vi "Shooter Control wPID.vi"() -> (7 "Robot Values Output":T1={"Robot Drive"={"Left Motor Power"=0.0, "Right Motor Power"=0.0, "Left Encoder Value"=0.0, "Right Encoder Value"=0.0, "High Gear?"=FALSE, "PTO?"=FALSE}, "Sensors"={"Gyro Angle"=0, "Recalibrate Gyro"=FALSE, "Reset Gyro"=FALSE, "Ultrasonic"=0.0}, "Shooter"={"Prep Wheels"=FALSE, "Shoot"=FALSE, "Left Shooter Wheel Speed"=0.0, "Wheels Moving"=FALSE, "Shooter Prepped"=FALSE, "Shooter RPS SP"=0.0, "Shooting?"=FALSE, "Left Shooter Wheel Power"=0.65, "Right Shooter Wheel Power"=0.0, "Acquisition Conveyor Power"=0.0, "Hopper Beater Bar Power"=0.0, "Filtered Left Shooter Speed"=0.0, "Acquisition Motor Power"=0.0, "Joystick Add"=0.0, "D-Pad Add"=0.0, "Shooter Use PID?"=FALSE}, "Robot States"={"Drive mode"="", "Alliance"=enum."Red", "Position"=enum."1"}, "Gear"={"Ejection Active"=FALSE}})   [LabVIEW 2016]
uses:
  Robot Values.ctl
  <vilib>/Rock Robotics/WPI/DriverStation/WPI_DriverStationAllianceInfo.ctl
  <vilib>/Rock Robotics/WPI/DriverStation/WPI_DriverStationPositionInfo.ctl
  <vilib>/Rock Robotics/Network Tables/NT Read Number.vi
  Robot Values.vi
  <vilib>/addons/control/pid/pid.llb/PID (DBL).vi
  LED Send Global.vi
  <vilib>/addons/control/pid/NI_PID_pid.lvlib
  <vilib>/ptbypt/NI_PtbyPt.lvlib
panel:
  in  "Feeder SP":dbl=0.88 format="%#_13g"
  out "Offset time":timestamp
  in  "Time Target In":dbl=0.6 caption="Time Target (s)"
  in  "Time Target Out":dbl caption="Time Target (s)"
  in  "Tolerance":dbl=2.0 format="%#_13g"
  in  "output range":cluster{"output high":dbl, "output low":dbl}={"output high"=0.049999999999999996, "output low"=-0.04999999999999999}
  in  "Agitate State":enum16{"In", "Out"}(ring)
  in  "Feeder Out SP":dbl=0.6
  in  "Feeder In SP":dbl=0.6
  out "Baseline Power":dbl=0.75 format="%#_13g"
  in  "Time Tolerance (s)":dbl=0.15 format="%#_13g"
  in  "PID gains":T4={"proportional gain (Kc)"=20.0, "integral time (Ti, min)"=0.010000000000000002, "derivative time (Td, min)"=0.0} {"derivative time (Td, min)" format="%.3f"; "integral time (Ti, min)" format="%.3f"; "proportional gain (Kc)" format="%.3f"}
  out "setpoint":dbl=39.0 format="%#_13g"
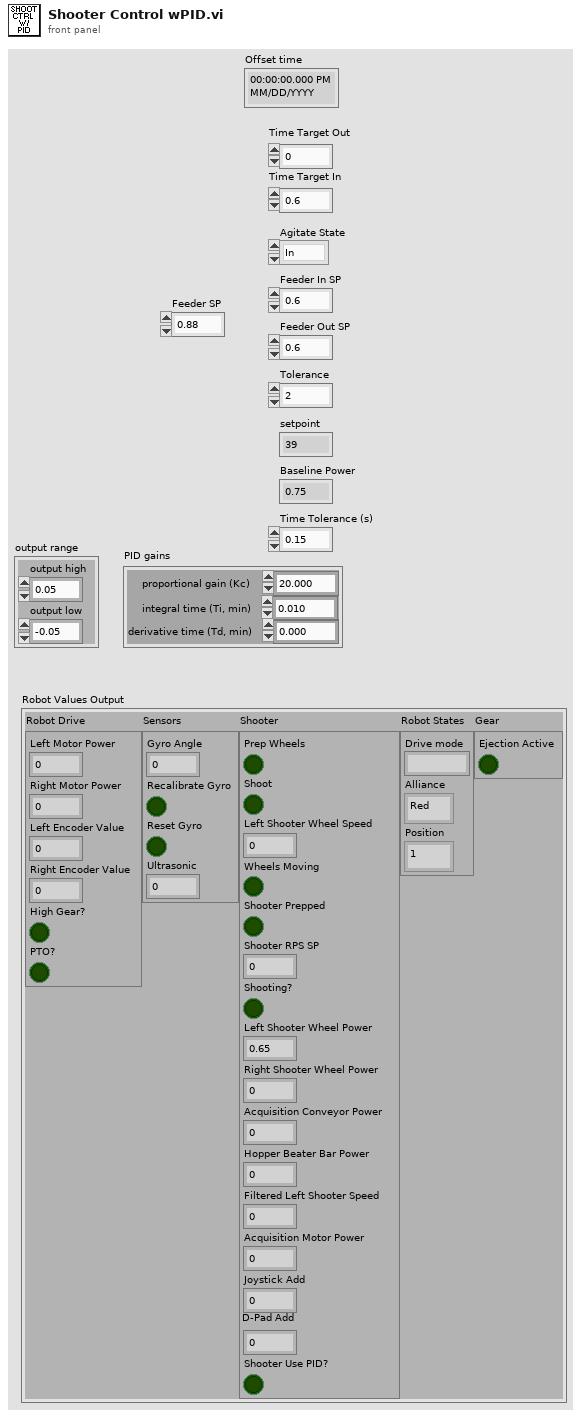
[diagram p1: front panel]
types:
  T1 = typedef "Robot Values.ctl" = cluster{"Robot Drive":cluster{"Left Motor Power":dbl, "Right Motor Power":dbl, "Left Encoder Value":dbl, "Right Encoder Value":dbl, "High Gear?":bool, "PTO?":bool}, "Sensors":cluster{"Gyro Angle":u16, "Recalibrate Gyro":bool, "Reset Gyro":bool, "Ultrasonic":dbl}, "Shooter":cluster{"Prep Wheels":bool, "Shoot":bool, "Left Shooter Wheel Speed":dbl, "Wheels Moving":bool, "Shooter Prepped":bool, "Shooter RPS SP":dbl, "Shooting?":bool, "Left Shooter Wheel Power":dbl, "Right Shooter Wheel Power":dbl, "Acquisition Conveyor Power":dbl, "Hopper Beater Bar Power":dbl, "Filtered Left Shooter Speed":dbl, "Acquisition Motor Power":dbl, "Joystick Add":dbl, "D-Pad Add":dbl, "Shooter Use PID?":bool}, "Robot States":cluster{"Drive mode":string, "Alliance":T2, "Position":T3}, "Gear":cluster{"Ejection Active":bool}}
  T2 = typedef "WPI_DriverStationAllianceInfo.ctl" = enum16{"Red", "Blue", "Invalid"}
  T3 = typedef "WPI_DriverStationPositionInfo.ctl" = enum16{"1", "2", "3"}
  T4 = cluster{"proportional gain (Kc)":dbl, "integral time (Ti, min)":dbl, "derivative time (Td, min)":dbl}
  T5 = typedef "LED Send Global.ctl" = cluster{"Underglow States":cluster{"RED":bool, "BLUE":bool}, "Hopper States":cluster{"No Shooter Power":bool, "1 RED":bool, "2 RED":bool, "3 RED":bool, "1 YEL 3 RED":bool, "2 YEL 3 RED":bool, "3 YEL 3 RED":bool, "1 GRN 3 YEL 3 RED":bool, "2 GRN 3 YEL 3 RED":bool, "3 GRN 3 YEL 3 RED":bool, "All GRN":bool, "Shooter w/Agitator":bool}, "License Plate States":cluster{"Auton States":cluster{"Do Nothing":bool, "Gear":bool, "Gear & Baseline":bool, "Gear & Shooter":bool, "Shooter":bool, "Shooter & Ball Dump":bool}, "Drive Train":cluster{"High Gear":bool, "Low Gear":bool}}, "Misc":cluster{"Pit/Demo":bool}, "Lights":cluster{"Underglow":string, "License Plate":string, "Hopper":string}}
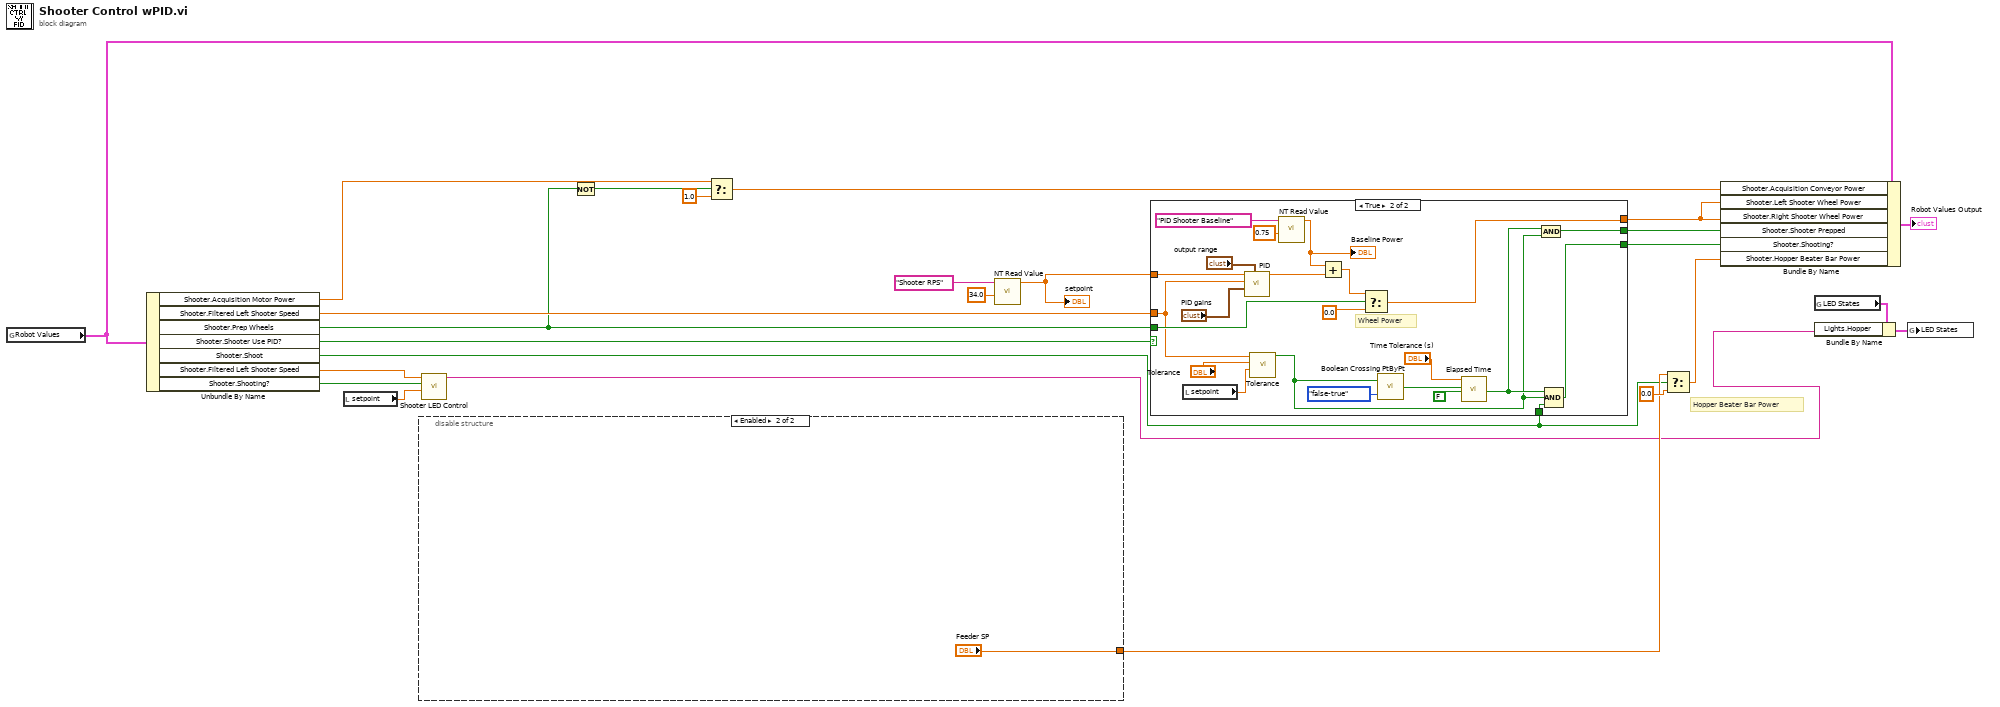
[diagram p0: block diagram]
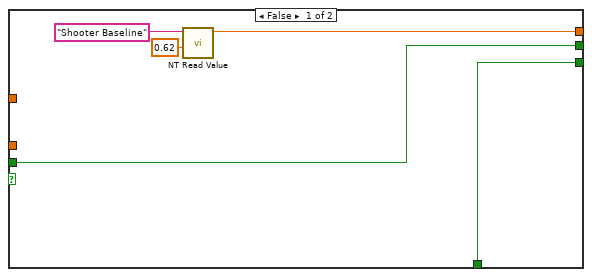
[diagram p2: hidden frame]
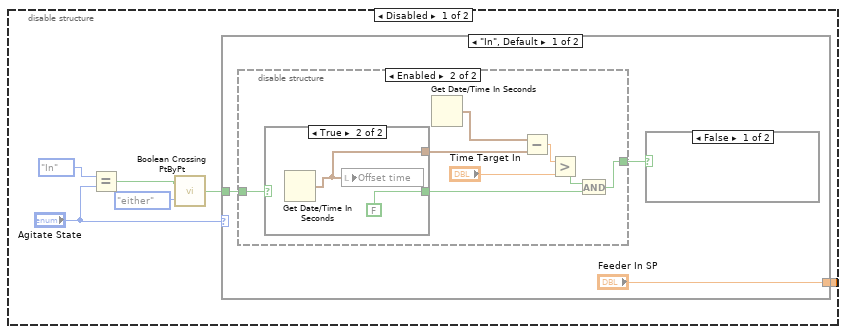
[diagram p3: hidden frame]
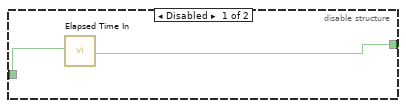
[diagram p4: hidden frame]
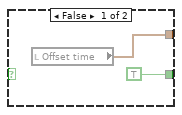
[diagram p5: hidden frame]
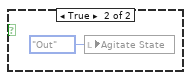
[diagram p6: hidden frame]
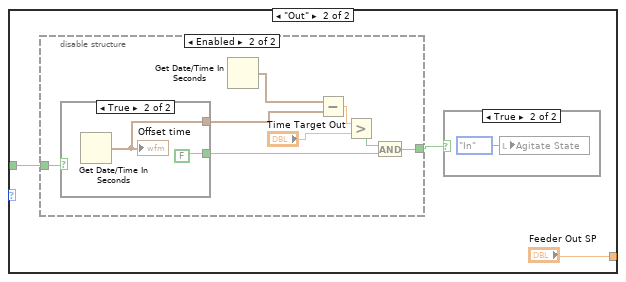
[diagram p7: hidden frame]
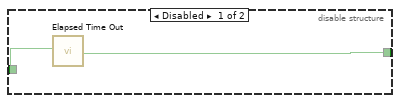
[diagram p8: hidden frame]
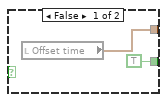
[diagram p9: hidden frame]
diagram:
  # "Hopper Beater Bar Power"
  n1 = global read "Robot Values.vi" "Robot Values"() -> (w23:T1)
  n2 = Unbundle By Name(w23) -> ("Shooter.Acquisition Motor Power"=w14:dbl, "Shooter.Filtered Left Shooter Speed"=w25:dbl, "Shooter.Prep Wheels"=w17:bool, "Shooter.Shooter Use PID?"=w1:bool, "Shooter.Shoot"=w11:bool, "Shooter.Filtered Left Shooter Speed"=w20:dbl, "Shooter.Shooting?"=w19:bool)
  n3 = local read "setpoint"() -> (w3:dbl)
  n4 = disable-structure shown="Enabled" {
    disable-tunnel: [w26 "Feeder SP"] -> w18
    frame Disabled {
      n5 = Equal?(x=enum16{"In", "Out"}."In" ("Agitate State"), y="Agitate State") -> (x = y?=w27:bool)
      n6 = call <vilib>:"Boolean Crossing PtByPt.vi"("direction"=enum16{"either", "false-true", "true-false"}."either", "input"=w27) -> ("crossing"=w28:bool)  [unwired: 1 in]
      n7 = case shown="\"In\", Default" "Agitate State" {
        tunnel: ["Feeder In SP" "Feeder Out SP"] -> w26
        tunnel: w28 -> [w32 w50]
        frame "In", Default {
          n8 = disable-structure shown="Enabled" {
            disable-tunnel: [w36 w38] -> w33
            disable-tunnel: w32 -> [w35 w40]
            frame Disabled {
              n9 = call "Elapsed Time In"("Reset"=w35) -> ("Time has Elapsed"=w36:bool)  [unwired: 11 in, 7 out]
            }
            frame Enabled {
              n10 = case shown="True" w40 {
                tunnel: [TRUE FALSE] -> w44
                tunnel: [w45 w47] -> w39
                frame False {
                  n11 = local read "Offset time"() -> (w45:timestamp)
                }
                frame True {
                  n12 = Get Date/Time In Seconds() -> (seconds since 1Jan1904=w47:timestamp)
                  n13 = local write "Offset time"(w47) -> ()
                }
              }
              n14 = Get Date/Time In Seconds() -> (seconds since 1Jan1904=w43:timestamp)
              n15 = Subtract(x=w43, y=w39) -> (x-y=w42:dbl)
              n16 = Greater?(x=w42, y="Time Target In") -> (0:w41:bool)
              n17 = And(x=w41, y=w44) -> (x .and. y?=w38:bool)
            }
          }
          n18 = case shown="False" w33 {
            frame False {
            }
            frame True {
              n19 = local write "Agitate State"(enum16{"In", "Out"}."Out" ("Agitate State")) -> ()
            }
          }
        }
        frame "Out" {
          n20 = disable-structure shown="Enabled" {
            disable-tunnel: [w54 w57] -> w51
            disable-tunnel: w50 -> [w53 w62]
            frame Disabled {
              n21 = call "Elapsed Time Out"("Reset"=w53) -> ("Time has Elapsed"=w54:bool)  [unwired: 11 in, 7 out]
            }
            frame Enabled {
              n22 = case shown="True" w62 {
                tunnel: [TRUE FALSE] -> w61
                tunnel: [w63 w65] -> w56
                frame False {
                  n23 = local read "Offset time"() -> (w63:timestamp)
                }
                frame True {
                  n24 = Get Date/Time In Seconds() -> (seconds since 1Jan1904=w65:timestamp)
                  "Offset time" <- w65
                }
              }
              n25 = Get Date/Time In Seconds() -> (seconds since 1Jan1904=w60:timestamp)
              n26 = Subtract(x=w60, y=w56) -> (x-y=w59:dbl)
              n27 = Greater?(x=w59, y="Time Target Out") -> (0:w58:bool)
              n28 = And(x=w58, y=w61) -> (x .and. y?=w57:bool)
            }
          }
          n29 = case shown="True" w51 {
            frame False {
            }
            frame True {
              n30 = local write "Agitate State"(enum16{"In", "Out"}."In" ("Agitate State")) -> ()
            }
          }
        }
      }
    }
    frame Enabled {
    }
  }
  n31 = call "Shooter LED Control.vi"("Current Shooter Speed"=w20, "Shooter Shooting"=w19, "Shooter SP"=w3) -> ("Shooter LED Send"=w5:string)  [unwired: 7 in]
  n32 = Not(x=w17) -> (.not. x?=w16:bool)
  n33 = Select(t=w14, s=w16, f=1.0) -> (s? t:f=w13:dbl)
  n34 = call-poly <vilib>:"NT Read Value.vi"("Default Value"=34.0, "Name"="Shooter RPS") -> ("Numeric"=w8:dbl)  [unwired: 8 in, 1 out]
  "setpoint" <- w8
  n35 = case shown="True" w1 {
    tunnel: [w72 w96] -> w24
    tunnel: w17 -> [w72 w95]
    tunnel: [w73 w94] -> w12
    tunnel: w11 -> [w73 w93]
    tunnel: w25 -> [_ w92]
    tunnel: w8 -> [_ w91]
    tunnel: [w69 w90] -> w7
    frame False {
      n36 = call-poly <vilib>:"NT Read Value.vi"("Default Value"=0.62, "Name"="Shooter Baseline") -> ("Numeric"=w69:dbl)  [unwired: 8 in, 1 out]
    }
    frame True {
      # "Wheel Power"
      n37 = local read "setpoint"() -> (w79:dbl)
      n38 = call-poly <vilib>:"PID.vi"("output range"="output range", "PID gains"="PID gains", "process variable"=w92, "setpoint"=w91) -> ("output"=w87:dbl)  [unwired: 6 in, 1 out]
      n39 = call "Tolerance.vi"("Setpoint"=w79, "Tolerance"="Tolerance", "Current Value"=w92) -> ("In Range?"=w77:bool)  [unwired: 8 in]
      n40 = call-poly <vilib>:"NT Read Value.vi"("Default Value"=0.75, "Name"="PID Shooter Baseline") -> ("Numeric"=w74:dbl)  [unwired: 8 in, 1 out]
      "Baseline Power" <- w74
      n41 = Add(x=w74, y=w87) -> (x+y=w88:dbl)
      n42 = Select(t=w88, s=w95, f=0.0) -> (s? t:f=w90:dbl)
      n43 = call <vilib>:"Boolean Crossing PtByPt.vi"("direction"=enum16{"either", "false-true", "true-false"}."false-true", "input"=w77) -> ("crossing"=w82:bool)  [unwired: 1 in]
      n44 = call "Elapsed Time"("Time Target (s)"="Time Tolerance (s)", "Reset"=w82, "Auto Reset"=FALSE) -> ("Time has Elapsed"=w78:bool)  [unwired: 9 in, 7 out]
      n45 = And(x=w78, y=w77) -> (x .and. y?=w96:bool)
      n46 = Compound Arithmetic op=AND(w78, w77, w93) -> (w94:bool)
    }
  }
  n47 = Select(t=w18, s=w11, f=0.0) -> (s? t:f=w21:dbl)
  n48 = Bundle By Name(cluster=w23, "Shooter.Acquisition Conveyor Power"=w13, "Shooter.Left Shooter Wheel Power"=w7, "Shooter.Right Shooter Wheel Power"=w7, "Shooter.Shooter Prepped"=w24, "Shooter.Shooting?"=w12, "Shooter.Hopper Beater Bar Power"=w21) -> (→"Robot Values Output":T1)
  n49 = global read "LED Send Global.vi" "LED States"() -> (w6:T5)
  n50 = Bundle By Name(cluster=w6, "Lights.Hopper"=w5) -> (w4:T5)
  n51 = global write "LED Send Global.vi" "LED States"(w4) -> ()
